vi "Run (ARGB).vi"(7 "OCR Level (Default: Word)":T5, 8 "error in (no error)":errorcluster, 10 "ARGB Image in":T4, 11 "Text Tesseract in":refnum<class "Text Tesseract.lvclass">) -> (0 "error out":errorcluster, 1 "Detections":T1[](array[typedef]), 2 "Detected Text":string, 3 "Text Tesseract":refnum<class "Text Tesseract.lvclass">)   [LabVIEW 2020, in "feature_detection.lvlib" / "Text Tesseract.lvclass"]
uses:
  Text Tesseract.lvclass
  OCR Level.ctl
  image/ARGB Image.ctl
  Detection Result.ctl
  Rectangle Corners.ctl
  common/Image Point (Integer).ctl
  Text Tesseract.lvclass/Text Tesseract.ctl
  image/Greyscale Image.ctl
  d21e2b8c-d7dd-47ce-9b78-18a6692dbbcb.vi
  <vilib>/Utility/error.llb/Error Cluster From Error Code.vi
  image/image.lvlib
  common/common.lvlib
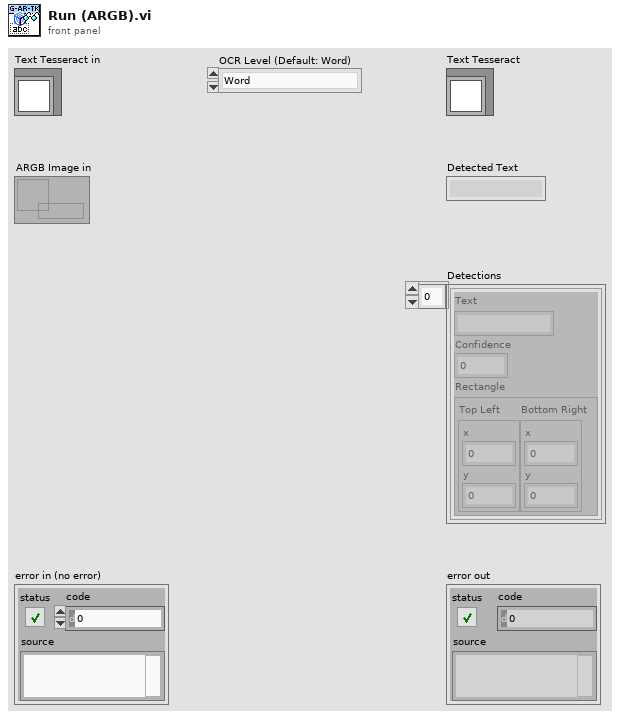
[diagram p1: front panel]
types:
  T1 = typedef "feature_detection.lvlib/Text Tesseract.lvclass/Detection Result.ctl" = cluster{"Text":string, "Confidence":sgl, "Rectangle":T2}
  T2 = typedef "feature_detection.lvlib/Text Tesseract.lvclass/Rectangle Corners.ctl" = cluster{"Top Left":T3, "Bottom Right":T3}
  T3 = typedef "common.lvlib/Image Point (Integer).ctl" = cluster{"x":i32, "y":i32}
  T4 = typedef "image.lvlib/ARGB Image.ctl" = refnum<data-value>
  T5 = typedef "feature_detection.lvlib/Text Tesseract.lvclass/OCR Level.ctl" = enum16{"Word", "Line"}
  T6 = typedef "image.lvlib/Greyscale Image.ctl" = refnum<data-value>
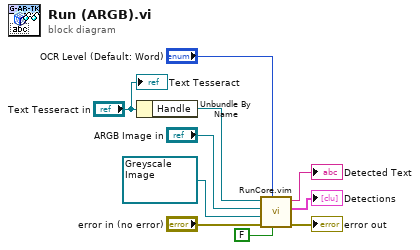
[diagram p0: block diagram]
diagram:
  n1 = Unbundle By Name("Text Tesseract in") -> ("Handle"=w10:refnum<data-value>)
  n2 = call "RunCore.vim"("Has Mask?"=FALSE, "OCR Level"="OCR Level (Default: Word)", "error in (no error)"="error in (no error)", "Mask"=T6 refnum ("Greyscale Image"), "Image in"="ARGB Image in", "Handle"=w10) -> ("error out"=→"error out":errorcluster, "Detections"=→"Detections":T1[], "Detected Text"=→"Detected Text":string)  [unwired: 3 in]
  "Text Tesseract" <- "Text Tesseract in"
